vi "FTW-SEQ-Construct.vi"(1 "Initial Sequence":string) -> (0 "Sequencer":refnum<class "FTW-Sequencer.lvclass">)   [LabVIEW 2012, in "FTW-Sequencer.lvclass"]
uses:
  FTW-Sequencer.lvclass
  FTW-Sequencer.lvclass/FTW-Sequencer.ctl
panel:
  # "Inputs"
  # "Outputs"
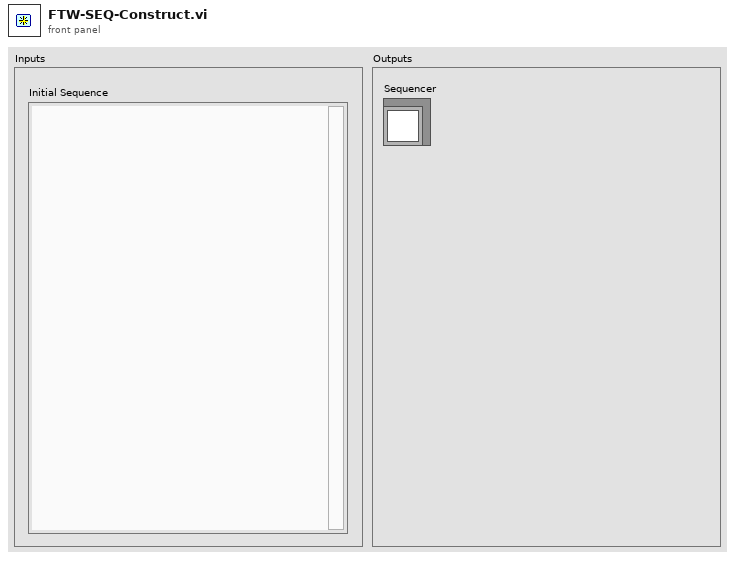
[diagram p1: front panel]
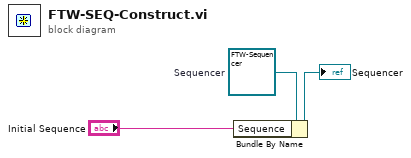
[diagram p0: block diagram]
diagram:
  w3 = refnum<class "FTW-Sequencer.lvclass"> refnum  # Sequencer
  n1 = Bundle By Name(cluster=w3, "Sequence"="Initial Sequence") -> (→"Sequencer":refnum<class "FTW-Sequencer.lvclass">)
